vi "xijk_combined_file_reader.vi"(8 "error in":errorcluster, 10 "channel":string, 11 "file path input":path) -> (0 "error out":errorcluster, 1 "file path out EM":path, 2 "file path out BS":path, 3 "file path out EX":path)   [LabVIEW 2009, in "xijk_combined_file.lvlib"]
uses:
  xijk_combined_file.lvlib
  <vilib>/Utility/file.llb/Read From Spreadsheet File (string).vi
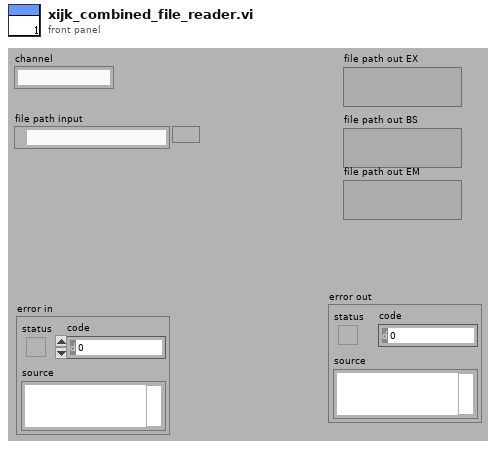
[diagram p1: front panel]
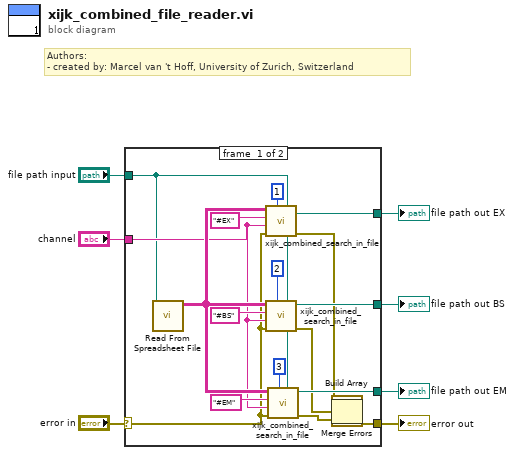
[diagram p0: block diagram]
diagram:
  # "Authors: \n- created by: Marcel van 't Hoff, University of Zurich, Switzerland"
  n1 = case shown="No Error" "error in" {
    selector: "error in" -> [w10 w26]
    tunnel: [w25 _] -> w7
    tunnel: [w24 _] -> w6
    tunnel: [w19 _] -> w5
    tunnel: "channel" -> [w18 _]
    tunnel: "file path input" -> [w14 _]
    tunnel: [w9 w26] -> w1
    frame #0 {
      n2 = call-poly <vilib>:"Read From Spreadsheet File.vi"("file path (dialog if empty)"=w14) -> ("all rows"=w23:string[][])  [unwired: 6 in, 4 out]
      n3 = call "xijk_combined_search_in_file.vi"("file path in"=w14, "index (col)"=1, "error in (no error)"=w10, "channel"=w18, "search input"="#EX" ("element"), "search 2D array"=w23) -> ("error out"=w13:errorcluster, "file path out"=w19:path)  [unwired: 4 in]
      n4 = call "xijk_combined_search_in_file.vi"("file path in"=w14, "index (col)"=2, "error in (no error)"=w10, "channel"=w18, "search input"="#BS" ("element"), "search 2D array"=w23) -> ("error out"=w12:errorcluster, "file path out"=w25:path)  [unwired: 4 in]
      n5 = call "xijk_combined_search_in_file.vi"("file path in"=w14, "index (col)"=3, "error in (no error)"=w10, "channel"=w18, "search input"="#EM" ("element"), "search 2D array"=w23) -> ("error out"=w11:errorcluster, "file path out"=w24:path)  [unwired: 4 in]
      n6 = Build Array(w13, w12, w11) -> (w8:errorcluster[])
      n7 = call <vilib>:"Merge Errors.vi"("error array in"=w8) -> ("error out"=w9:errorcluster)  [unwired: 6 in]
    }
    frame #1 {
    }
  }
  "file path out EX" <- w5
  "file path out BS" <- w7
  "file path out EM" <- w6
  "error out" <- w1
